vi "Get Coordinates.vi"(8 "error in (no error)":errorcluster, 9 "Plot ID":i32, 11 "3D Quiver.lvclass in":refnum<class "3D Quiver.lvclass">) -> (0 "error out":errorcluster, 1 "Coordinates System":enum16{"Cartesian", "Cylindrical", "Spherical"}(ring), 3 "3D Quiver.lvclass out":refnum<class "3D Quiver.lvclass">)   [LabVIEW 2020, in "3D Quiver.lvclass"]
uses:
  <vilib>/Math Plots/3D Math Plots/3D Quiver/3D Quiver/3D Quiver.lvclass
  <vilib>/Math Plots/3D Math Plots/3D Quiver/3D Quiver/3D Quiver.lvclass/3D Quiver.ctl
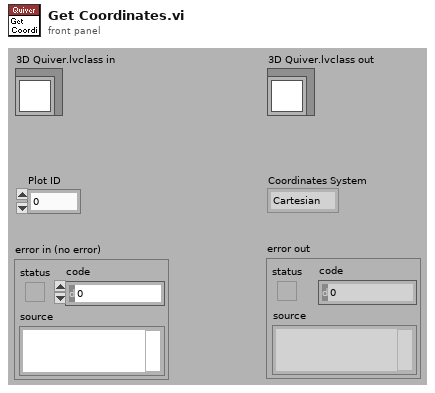
[diagram p1: front panel]
types:
  T1 = typedef "3D Quiver.lvclass/3D Quiver Property Array.ctl" = T2[]
  T2 = typedef "3D Quiver.lvclass/3D Quiver Property.ctl" = cluster{"General Property":cluster{"Plot Name":string, "Coordinate System":enum16{"Cartesian", "Cylindrical", "Spherical"}, "Opacity":sgl}, "Projection Property":cluster{"Draw XY":bool, "Draw YZ":bool, "Draw XZ":bool}, "Plot Property":cluster{"Line Style":T3, "Line Width":sgl, "Line Color":u32, "Antialiasing":bool, "Color Ramp Cluster":T4}, "Quiver Property":cluster{"Quvier Mode":enum16{"Quiver", "Quiver with surface"}, "Quiver Size":sgl, "Quiver Length":sgl}}
  T3 = typedef "3D Plot.lvclass/Line Type.ctl" = enum16{"None", "Solid", "Dash", "Dot", "Dash Dot"}
  T4 = typedef "3D Plot.lvclass/Color Ramp Cluster.ctl" = cluster{"Color Ramp Style":enum16{"None", "Shaded", "Color spectrum", "Grey scale", "Custom"}, "Color Ramp Array":u32[], "Color Ramp Index":i32[], "Interpolate?":bool, "Logarithm?":bool}
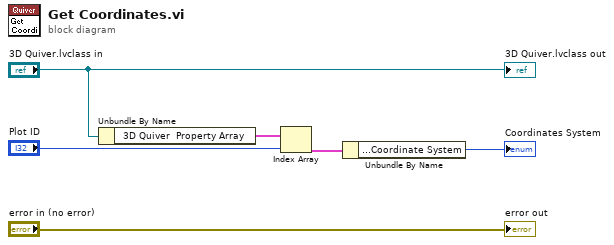
[diagram p0: block diagram]
diagram:
  n1 = Unbundle By Name("3D Quiver.lvclass in") -> ("3D Quiver  Property Array"=w6:T1)
  n2 = Index Array(array=w6, index="Plot ID") -> (element=w5:T2)
  n3 = Unbundle By Name(w5) -> ("General Property.Coordinate System"=→"Coordinates System":enum16{"Cartesian", "Cylindrical", "Spherical"})
  "3D Quiver.lvclass out" <- "3D Quiver.lvclass in"
  "error out" <- "error in (no error)"
